vi "LoadDAQSettings.vi"(2 "error in":errorcluster, 3 "DAQ Card/Channels":i32[](array[numeric]), 4 "Current ExpState IN":T5={"error"={"status"=FALSE, "code"=0, "source"=""}, "Digitizer DAQmx Tasks"={"TaskArray"=[]}, "Digitizer Settings"={"Channel Settings"=[], "Card Settings"=[]}, "Synchronization Settings"={"Synchronizer"="", "source terminal"=""}, "Digitizer Data"=[], "Next Shot#"="", "System Message"="", "User Shot Notes"="", "Timing Settings"={"Timing Card Settings"=[], "Timing Channel Settings"=[]}, "Timing Tasks"={"TaskArray"=[]}, "Tree"="", "Time Card/Channels"=[2, 8], "DAQ Card/Channels"=[3, 8], "Program Version"="", "RIO Settings"={"Channel Settings"=[], "Card Settings"=[]}, "RIO References"={"Reference Array"=[]}} {"RIO Settings"."Card Settings"."Sample Rate" format="%#_3p"; "Timing Settings"."Timing Channel Settings"."FrontPanelTime" format="%.3p"; "Timing Settings"."Timing Channel Settings"."Pulse width (s)" format="%.3p"; "Timing Settings"."Timing Channel Settings"."Delay (s)" format="%.3p"; "Digitizer Settings"."Card Settings"."Global Edge Type" items=["Rising"=10280, "Falling"=10171]; "Digitizer Settings"."Card Settings"."Sample Rate" format="%#_3p"}, 5 "Tree DVR In":refnum<data-value>) -> (0 "error out":errorcluster, 1 "Digitizer Settings":T4 {"Card Settings"."Global Edge Type" items=["Rising"=10280, "Falling"=10171]; "Card Settings"."Sample Rate" format="%#_3p"})   [LabVIEW 2014]
uses:
  Controls/ExperimentStateCluster.ctl
  Controls/DigitizerSettingsChannelSettings.ctl
  Controls/DigitizerSettingsCardSettingsArray.ctl
  Controls/DigitizerSettingsCardSettings.ctl
  Controls/TimingSettings.ctl
  Controls/TimingCardSettings.ctl
  Controls/TimingChannelSettings.ctl
  Controls/RIOSettingsExperimentStateCluster.ctl
  Controls/RIOSettingsChannelSettings.ctl
  Controls/RIOSettingsCardSettingsArray.ctl
  Controls/RIOSettingsCardSettings.ctl
  <vilib>/userdefined/High Color/nirio_resource_hc.ctl
  <vilib>/MDSplus/Classes/Tree_Class/Tree.lvclass
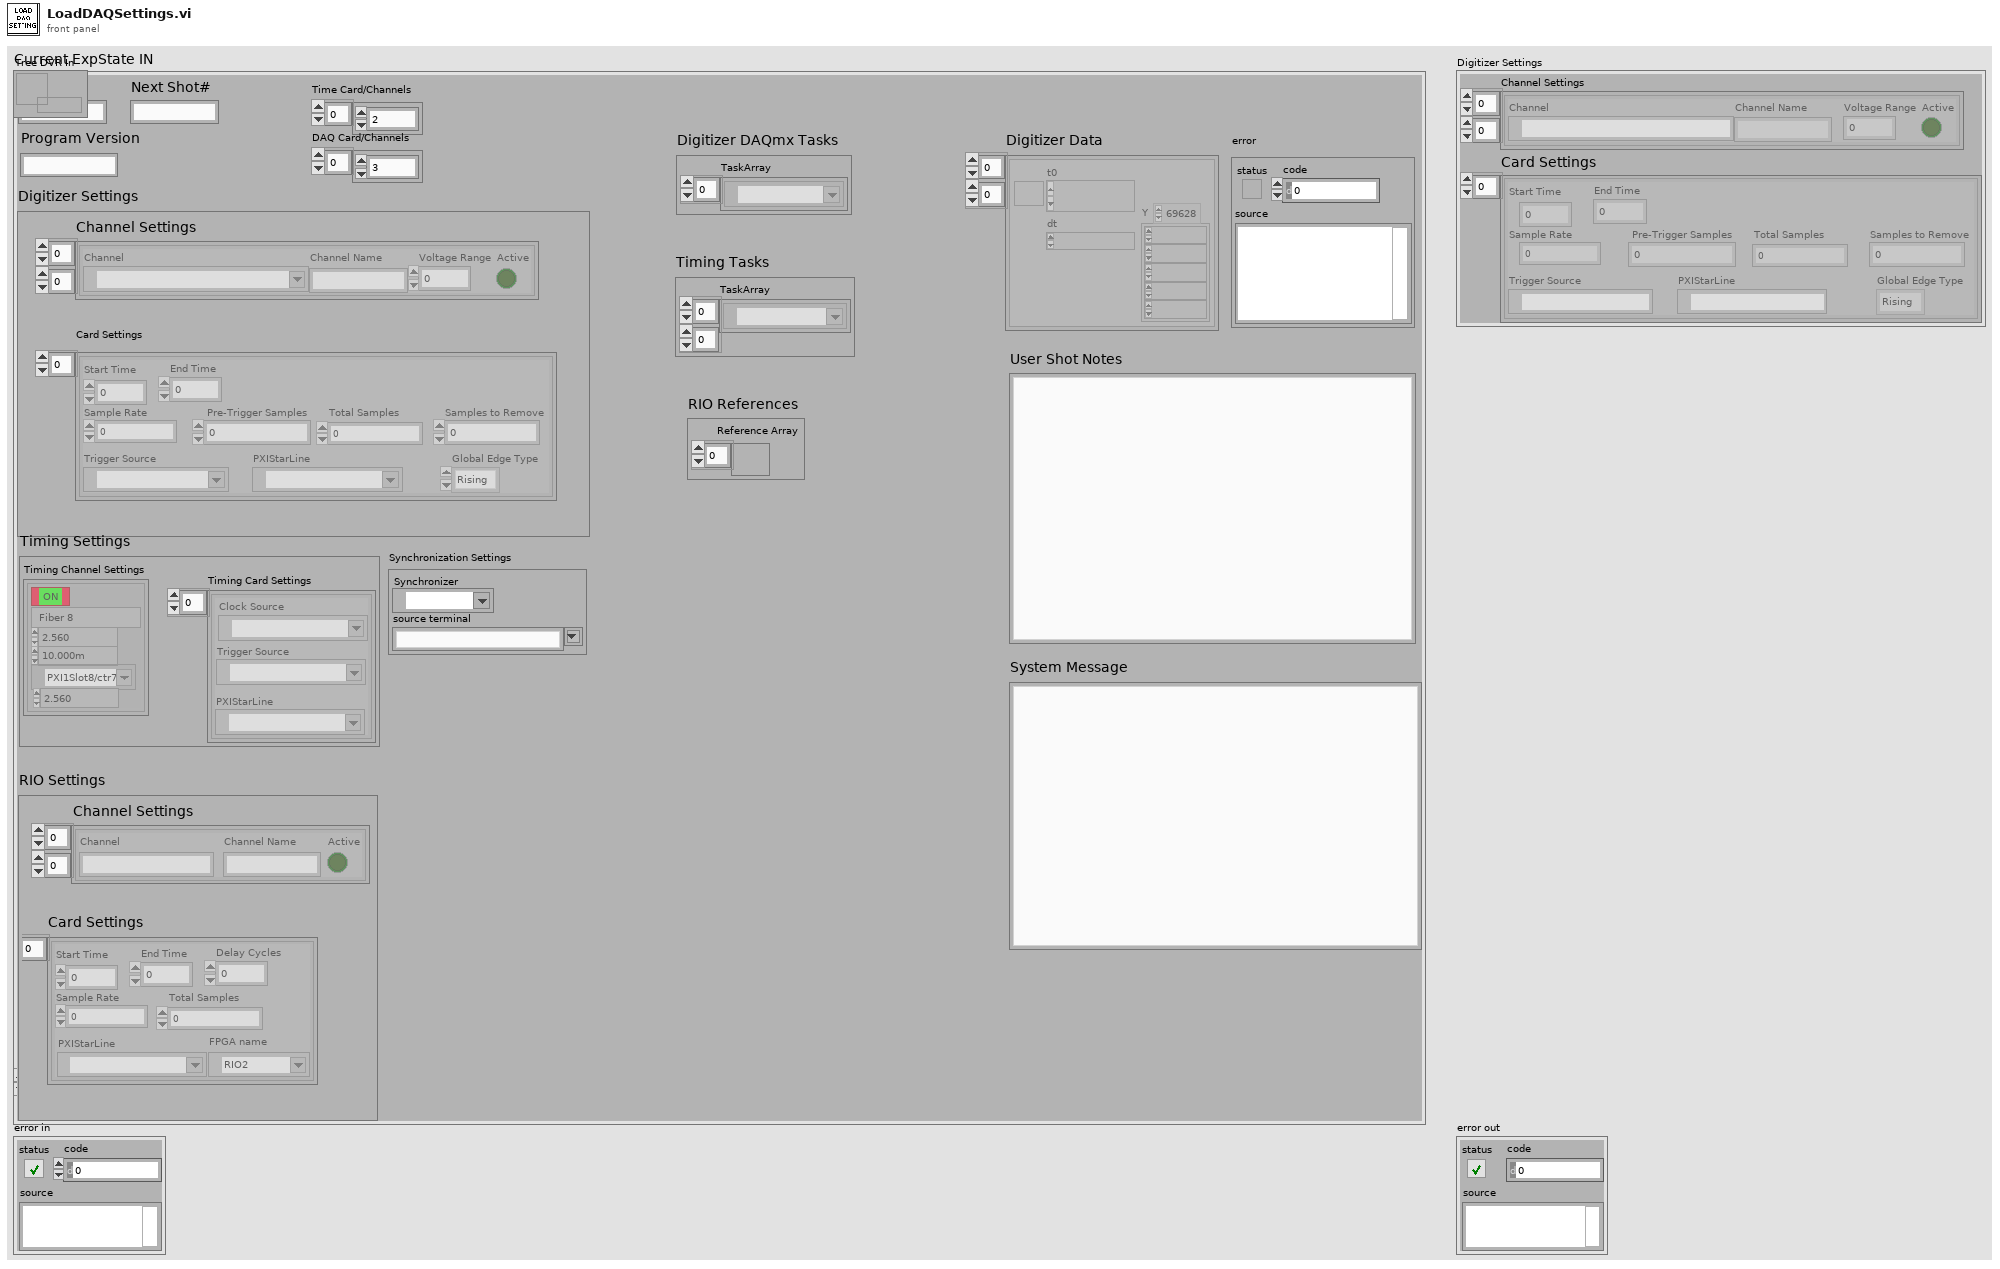
[diagram p1: front panel]
types:
  T1 = typedef "DigitizerSettingsChannelSettings.ctl" = cluster{"Channel":tag, "Channel Name":string, "Voltage Range":dbl, "Active":bool}
  T2 = typedef "DigitizerSettingsCardSettingsArray.ctl" = T3[]
  T3 = typedef "DigitizerSettingsCardSettings.ctl" = cluster{"Start Time":dbl, "End Time":dbl, "Sample Rate":dbl, " Pre-Trigger Samples":u32, "Total Samples":i32, "Samples to Remove":u32, "Trigger Source":tag, "Global Edge Type":i32, "PXIStarLine":tag}
  T4 = cluster{"Channel Settings":T1[][], "Card Settings":T2}
  T5 = typedef "ExperimentStateCluster.ctl" = cluster{"error":errorcluster, "Digitizer DAQmx Tasks":cluster{"TaskArray":refnum<k21>[]}, "Digitizer Settings":cluster{"Channel Settings":T1[][], "Card Settings":T2}, "Synchronization Settings":cluster{"Synchronizer":refnum<k15>, "source terminal":string}, "Digitizer Data":waveform(dbl)[][], "Next Shot#":string, "System Message":string, "User Shot Notes":string, "Timing Settings":T6, "Timing Tasks":cluster{"TaskArray":refnum<k21>[][]}, "Tree":string, "Time Card/Channels":i32[], "DAQ Card/Channels":i32[], "Program Version":string, "RIO Settings":T9, "RIO References":cluster{"Reference Array":refnum<k20>[]}}
  T6 = typedef "TimingSettings.ctl" = cluster{"Timing Card Settings":T7[], "Timing Channel Settings":T8[][]}
  T7 = typedef "TimingCardSettings.ctl" = cluster{"Trigger Source":tag, "Clock Source":tag, "PXIStarLine":tag}
  T8 = typedef "TimingChannelSettings.ctl" = cluster{"Delay (s)":dbl, "Pulse width (s)":dbl, "Active":bool, "Channel Name":string, "counter":tag, "FrontPanelTime":dbl}
  T9 = typedef "RIOSettingsExperimentStateCluster.ctl" = cluster{"Channel Settings":T10[][], "Card Settings":T11}
  T10 = typedef "RIOSettingsChannelSettings.ctl" = cluster{"Channel Name":string, "Active":bool, "Channel":string}
  T11 = typedef "RIOSettingsCardSettingsArray.ctl" = T12[]
  T12 = typedef "RIOSettingsCardSettings.ctl" = cluster{"Start Time":dbl, "End Time":dbl, "Sample Rate":dbl, "Total Samples":u64, "PXIStarLine":tag, "Delay Cycles":u64, "FPGA name":T13}
  T13 = typedef "nirio_resource_hc.ctl" = tag
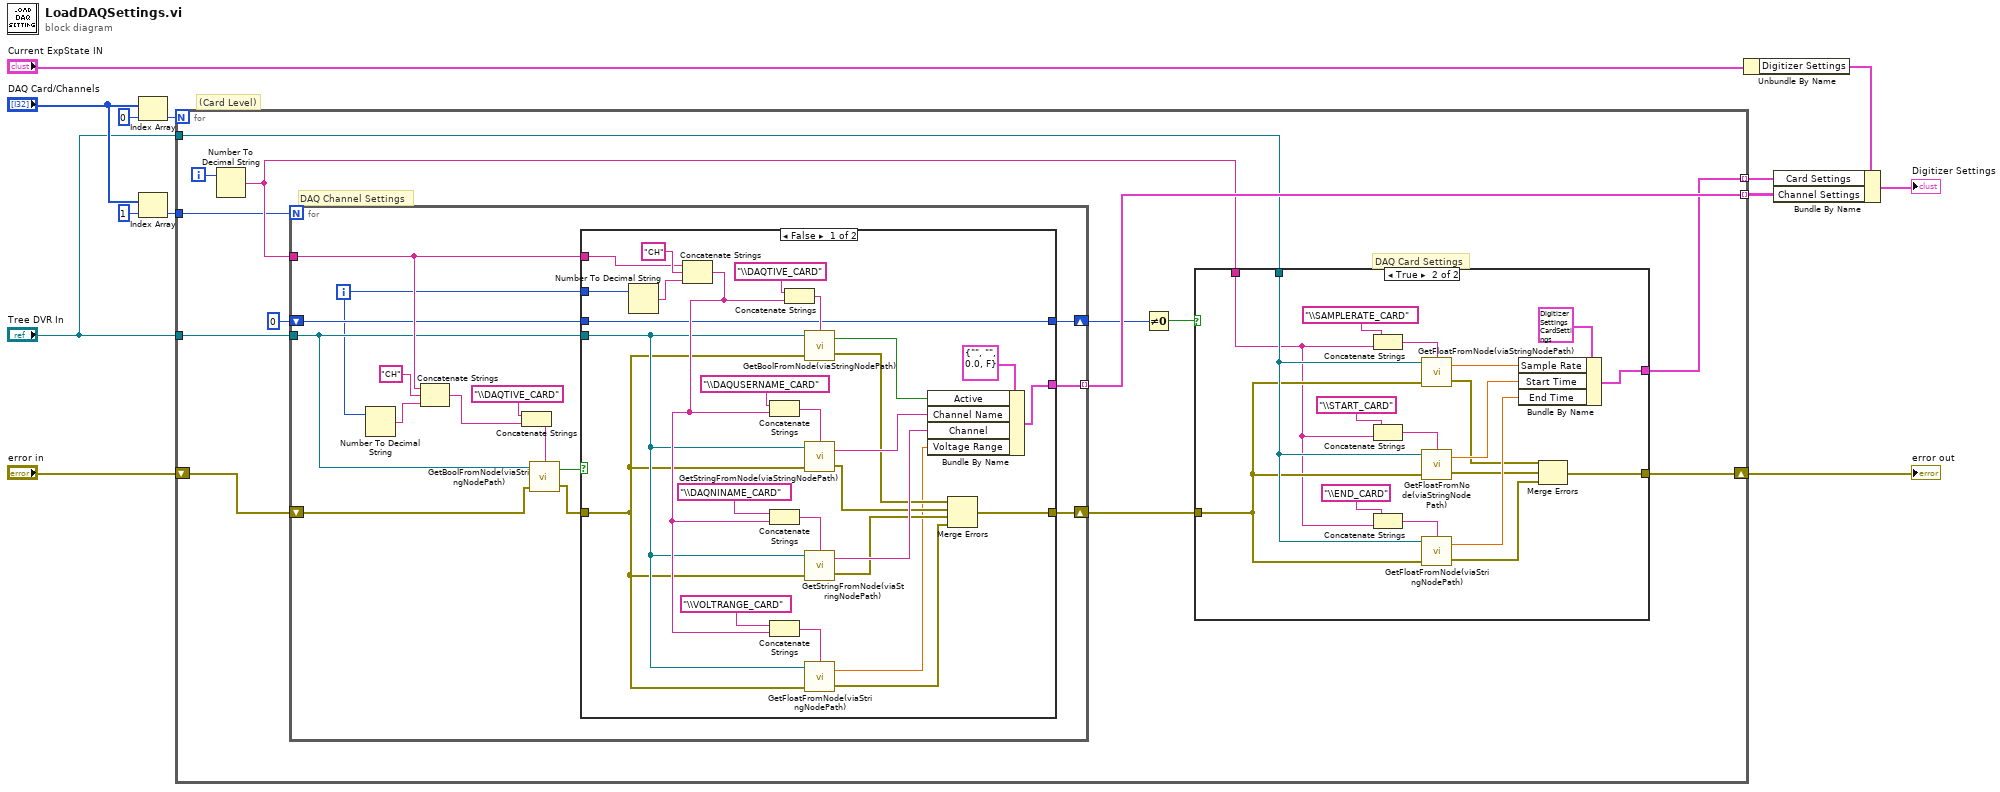
[diagram p0: block diagram]
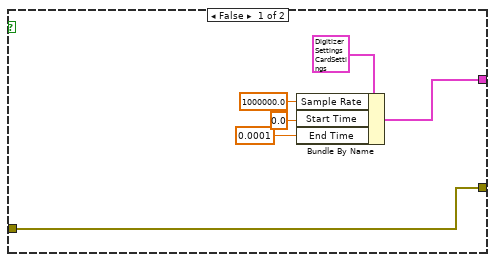
[diagram p2: hidden frame]
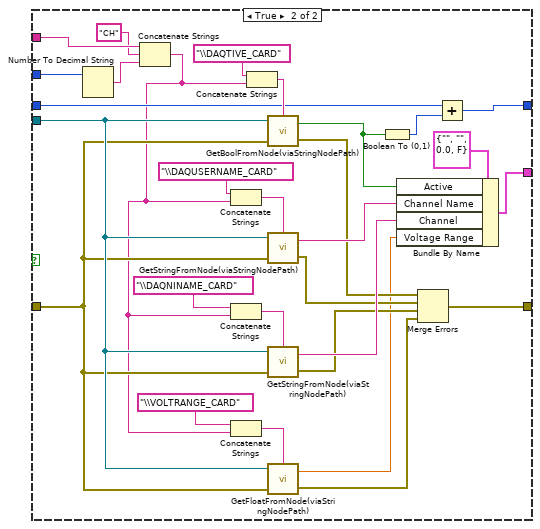
[diagram p3: hidden frame]
diagram:
  # "(Card Level)"
  n1 = Index Array(array="DAQ Card/Channels", index=0) -> (element=w11:i32)
  n2 = Index Array(array="DAQ Card/Channels", index=1) -> (element=w13:i32)
  n3 = for {
    N: w11 -> [_]
    tunnel: "Tree DVR In" -> [w25]
    shift-right: [w20] -> w4
    shift-left: "error in" -> [w15]
    tunnel: "Tree DVR In" -> [w22]
    tunnel: [w24] -> w2 mode=indexing
    tunnel: w13 -> [w16]
    tunnel: [w19] -> w3 mode=indexing
    i -> [w26]
    # "DAQ Card Settings"
    # "DAQ Channel Settings"
    n4 = Number To Decimal String(number=w26) -> (decimal integer string=w18:string)  [unwired: 1 in]
    n5 = for {
      N: w16 -> [_]
      tunnel: w25 -> [w52]
      tunnel: [w65] -> w24 mode=indexing
      tunnel: w18 -> [w62]
      shift-right: [w63] -> w21
      shift-left: w15 -> [w54]
      shift-right: [w64] -> w23
      shift-left: 0 -> [w61]
      i -> [w51]
      n6 = Number To Decimal String(number=w51) -> (decimal integer string=w59:string)  [unwired: 1 in]
      n7 = Concatenate Strings(w62, "CH" ("string"), w59) -> (w57:string)
      n8 = Concatenate Strings("\\DAQTIVE_CARD" ("string"), w57) -> (w56:string)
      n9 = call "GetBoolFromNode(viaStringNodePath).vi"("Path"=w56, "error in"=w54, "Tree DVR in"=w52) -> ("error out"=w53:errorcluster, "Bool Out"=w55:bool)  [unwired: 1 in]
      n10 = case shown="False" w55 {
        tunnel: w52 -> [w69 w113]
        tunnel: w53 -> [w68 w112]
        tunnel: [w67 w105] -> w63
        tunnel: [w72 w104] -> w65
        tunnel: w61 -> [w66 w101]
        tunnel: [w66 w99] -> w64
        tunnel: w62 -> [w71 w98]
        tunnel: w51 -> [w70 w93]
        frame False {
          n11 = Number To Decimal String(number=w70) -> (decimal integer string=w76:string)  [unwired: 1 in]
          n12 = Concatenate Strings(w71, "CH" ("string"), w76) -> (w74:string)
          n13 = Concatenate Strings("\\DAQUSERNAME_CARD" ("string"), w74) -> (w88:string)
          n14 = Concatenate Strings("\\DAQNINAME_CARD" ("string"), w74) -> (w87:string)
          n15 = Concatenate Strings("\\VOLTRANGE_CARD" ("string"), w74) -> (w86:string)
          n16 = Concatenate Strings("\\DAQTIVE_CARD" ("string"), w74) -> (w89:string)
          n17 = call "GetBoolFromNode(viaStringNodePath).vi"("Path"=w89, "error in"=w68, "Tree DVR in"=w69) -> ("error out"=w82:errorcluster, "Bool Out"=w77:bool)  [unwired: 1 in]
          n18 = call "GetStringFromNode(viaStringNodePath).vi"("Path"=w88, "error in"=w68, "Tree DVR in"=w69) -> ("error out"=w81:errorcluster, "String out"=w84:string)  [unwired: 1 in]
          n19 = call "GetStringFromNode(viaStringNodePath).vi"("Path"=w87, "error in"=w68, "Tree DVR in"=w69) -> ("error out"=w80:errorcluster, "String out"=w83:string)  [unwired: 1 in]
          n20 = call "GetFloatFromNode(viaStringNodePath).vi"("Path"=w86, "error in"=w68, "Tree DVR in"=w69) -> ("error out"=w79:errorcluster, "Float64"=w78:dbl)  [unwired: 1 in]
          n21 = Bundle By Name(cluster=T1 {"Channel"="", "Channel Name"="", "Voltage Range"=0.0, "Active"=FALSE} ("Channel Setting"), "Active"=w77, "Channel Name"=w84, "Channel"=w83, "Voltage Range"=w78) -> (w72:T1)
          n22 = Merge Errors(w82, w81, w80, w79) -> (w67:errorcluster)
        }
        frame True {
          n23 = Number To Decimal String(number=w93) -> (decimal integer string=w97:string)  [unwired: 1 in]
          n24 = Concatenate Strings(w98, "CH" ("string"), w97) -> (w95:string)
          n25 = Concatenate Strings("\\DAQUSERNAME_CARD" ("string"), w95) -> (w117:string)
          n26 = Concatenate Strings("\\DAQNINAME_CARD" ("string"), w95) -> (w116:string)
          n27 = Concatenate Strings("\\VOLTRANGE_CARD" ("string"), w95) -> (w115:string)
          n28 = Concatenate Strings("\\DAQTIVE_CARD" ("string"), w95) -> (w118:string)
          n29 = call "GetBoolFromNode(viaStringNodePath).vi"("Path"=w118, "error in"=w112, "Tree DVR in"=w113) -> ("error out"=w109:errorcluster, "Bool Out"=w102:bool)  [unwired: 1 in]
          n30 = call "GetStringFromNode(viaStringNodePath).vi"("Path"=w117, "error in"=w112, "Tree DVR in"=w113) -> ("error out"=w108:errorcluster, "String out"=w111:string)  [unwired: 1 in]
          n31 = call "GetStringFromNode(viaStringNodePath).vi"("Path"=w116, "error in"=w112, "Tree DVR in"=w113) -> ("error out"=w107:errorcluster, "String out"=w110:string)  [unwired: 1 in]
          n32 = call "GetFloatFromNode(viaStringNodePath).vi"("Path"=w115, "error in"=w112, "Tree DVR in"=w113) -> ("error out"=w106:errorcluster, "Float64"=w103:dbl)  [unwired: 1 in]
          n33 = Boolean To (0,1)(Boolean=w102) -> (0, 1=w100:i16)
          n34 = Bundle By Name(cluster=T1 {"Channel"="", "Channel Name"="", "Voltage Range"=0.0, "Active"=FALSE} ("Channel Setting"), "Active"=w102, "Channel Name"=w111, "Channel"=w110, "Voltage Range"=w103) -> (w104:T1)
          n35 = Merge Errors(w109, w108, w107, w106) -> (w105:errorcluster)
          n36 = Add(x=w101, y=w100) -> (x+y=w99:i32)
        }
      }
    }
    n37 = Not Equal To 0?(x=w23) -> (x != 0?=w14:bool)
    n38 = case shown="True" w14 {
      tunnel: w22 -> [_ w50]
      tunnel: w21 -> [w27 w49]
      tunnel: [w27 w48] -> w20
      tunnel: [w28 w47] -> w19
      tunnel: w18 -> [_ w46]
      frame False {
        n39 = Bundle By Name(cluster=T3 {"Start Time"=0.0, "End Time"=0.0, "Sample Rate"=0.0, " Pre-Trigger Samples"=0, "Total Samples"=0, "Samples to Remove"=0, "Trigger Source"="", "Global Edge Type"=10280, "PXIStarLine"=""} ("Card Setting"), "Sample Rate"=1000000.0, "Start Time"=0.0, "End Time"=0.0001) -> (w28:T3)
      }
      frame True {
        n40 = Concatenate Strings("\\SAMPLERATE_CARD" ("string"), w46) -> (w44:string)
        n41 = Concatenate Strings("\\START_CARD" ("string"), w46) -> (w40:string)
        n42 = Concatenate Strings("\\END_CARD" ("string"), w46) -> (w43:string)
        n43 = call "GetFloatFromNode(viaStringNodePath).vi"("Path"=w44, "error in"=w49, "Tree DVR in"=w50) -> ("error out"=w36:errorcluster, "Float64"=w39:dbl)  [unwired: 1 in]
        n44 = call "GetFloatFromNode(viaStringNodePath).vi"("Path"=w40, "error in"=w49, "Tree DVR in"=w50) -> ("error out"=w35:errorcluster, "Float64"=w38:dbl)  [unwired: 1 in]
        n45 = call "GetFloatFromNode(viaStringNodePath).vi"("Path"=w43, "error in"=w49, "Tree DVR in"=w50) -> ("error out"=w34:errorcluster, "Float64"=w37:dbl)  [unwired: 1 in]
        n46 = Bundle By Name(cluster=T3 {"Start Time"=0.0, "End Time"=0.0, "Sample Rate"=0.0, " Pre-Trigger Samples"=0, "Total Samples"=0, "Samples to Remove"=0, "Trigger Source"="", "Global Edge Type"=10280, "PXIStarLine"=""} ("Card Setting"), "Sample Rate"=w39, "Start Time"=w38, "End Time"=w37) -> (w47:T3)
        n47 = Merge Errors(w36, w35, w34) -> (w48:errorcluster)
      }
    }
  }
  "error out" <- w4
  n48 = Unbundle By Name("Current ExpState IN") -> ("Digitizer Settings"=w8:T4)
  n49 = Bundle By Name(cluster=w8, "Card Settings"=w3, "Channel Settings"=w2) -> (→"Digitizer Settings":T4)
